vi "Pose2D_subscriber.vi"() -> ()   [LabVIEW 2014]
panel:
  out "theta":dbl
  out "y":dbl
  out "x":dbl
  in  "停止":bool
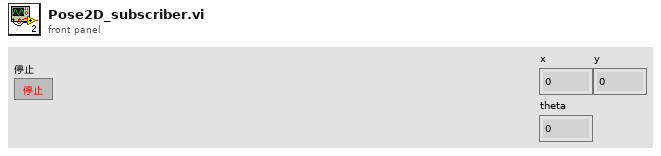
[diagram p1: front panel]
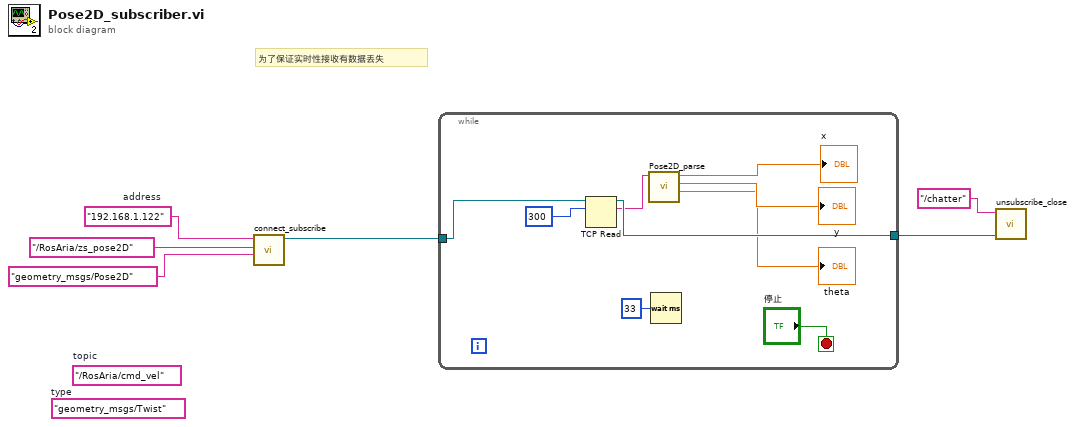
[diagram p0: block diagram]
diagram:
  (unwired) "geometry_msgs/Twist"  # type
  (unwired) "/RosAria/cmd_vel"  # topic
  w6 = "192.168.1.122"  # address
  # "为了保证实时性接收有数据丢失"
  n1 = call "connect_subscribe.vi"("type"="geometry_msgs/Pose2D", "topic"="/RosAria/zs_pose2D", "address"=w6) -> ("连接ID输出"=w5:refnum<k5>)  [unwired: 7 in, 1 out]
  n2 = while {
    tunnel: [w15] -> w2
    tunnel: w5 -> [w12]
    stop <- "停止" stop-if-true
    n3 = TCP Read(connection ID=w12, bytes to read=300 ("读取的字节")) -> (connection ID out=w15:refnum<k5>, data out=w11:string)  [unwired: 3 in, 1 out]
    n4 = call "Pose2D_parse.vi"("字符串"=w11) -> ("theta"=→"theta":dbl, "y"=→"y":dbl, "x"=→"x":dbl)  [unwired: 8 in]
    n5 = Wait (ms)(milliseconds to wait=u32 33 ("等待时间（毫秒）")) -> ()  [unwired: 1 out]
  }
  n6 = call "unsubscribe_close.vi"("连接ID"=w2, "topic"="/chatter") -> ()  [unwired: 10 in]
